vi "ROS Init websock.vi"(6 "topic":cluster{"Topic to write":string, "type":string}={"Topic to write"="rio/odom", "type"="sterowanie/velocities"}, 10 "rosbridge port":u16, 11 "rosbridge  IP":string) -> (3 "output":T1, 4 "Topic to write":string)   [LabVIEW 2015]
uses:
  <vilib>/MediaMongrels Ltd/WebSockets/WebSockets/WebSockets.lvlib
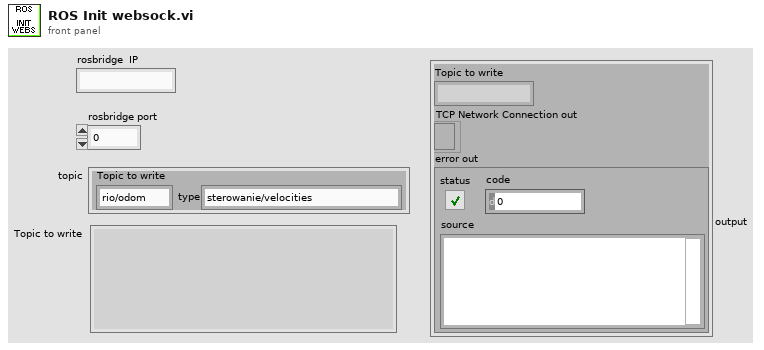
[diagram p1: front panel]
types:
  T1 = cluster{"Topic to write":string, "TCP Network Connection out":refnum<k5>, "error out":errorcluster}
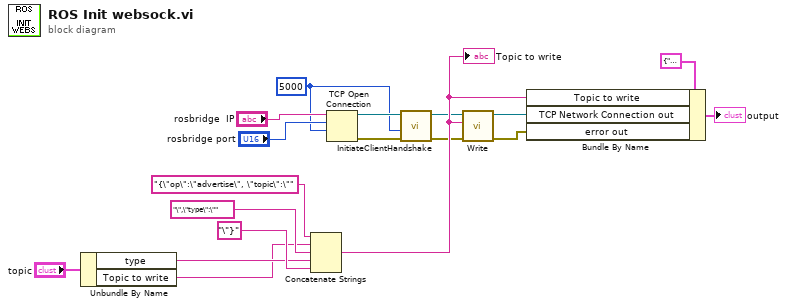
[diagram p0: block diagram]
diagram:
  w3 = 5000 ("timeout ms (60000)")
  n1 = Unbundle By Name("topic") -> ("type"=w12:string, "Topic to write"=w7:string)
  n2 = Concatenate Strings("{\"op\":\"advertise\", \"topic\":\"", w7, "\",\"type\":\"", w12, "\"}") -> (w6:string)
  "Topic to write" <- w6
  n3 = TCP Open Connection(address="rosbridge  IP", remote port or service name="rosbridge port", timeout ms (60000)=w3) -> (connection ID=w5:refnum<k5>, error out=w4:errorcluster)  [unwired: 2 in]
  n4 = call <vilib>:"InitiateClientHandshake.vi"("error in (no error)"=w4, "timeout ms (5000)"=w3, "WebSocket Connection in"=w5) -> ("error out"=w1:errorcluster, "WebSocket Connection out"=w2:refnum<k5>)  [unwired: 6 in, 1 out]
  n5 = call <vilib>:"Write.vi"("error in (no error)"=w1, "Data"=w6, "WebSocket Connection in"=w2) -> ("error out"=w9:errorcluster, "WebSocket Connection out"=w11:refnum<k5>)  [unwired: 7 in]
  n6 = Bundle By Name(cluster=T1 {"Topic to write"="", "TCP Network Connection out"=refnum, "error out"={"status"=FALSE, "code"=0, "source"=""}} ("input cluster"), "Topic to write"=w6, "TCP Network Connection out"=w11, "error out"=w9) -> (→"output":T1)
